vi "subvi_jenoptik_monotonize.vi"(1 "Array":dbl[](array[numeric]) format="%.2f") -> (0 "phase":dbl[](array[numeric]) format="%.2f")   [LabVIEW 2020]
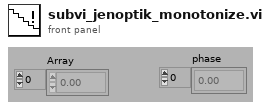
[diagram p1: front panel]
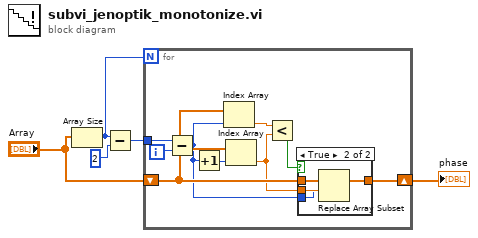
[diagram p0: block diagram]
diagram:
  n1 = Array Size(array="Array") -> (size(s)=w3:i32)
  n2 = Subtract(x=w3, y=2) -> (x-y=w2:i32)
  n3 = for {
    N: w3 -> [_]
    shift-right: [w14] -> w4
    shift-left: "Array" -> [w10]
    tunnel: w2 -> [w13]
    i -> [w12]
    n4 = Subtract(x=w13, y=w12) -> (x-y=w6:i32)
    n5 = Increment(x=w6) -> (x+1=w11:i32)
    n6 = Index Array(array=w10, index=w6) -> (element=w9:dbl)
    n7 = Index Array(array=w10, index=w11) -> (element=w7:dbl)
    n8 = Less?(x=w9, y=w7) -> (x < y?=w8:bool)
    n9 = case shown="True" w8 {
      tunnel: [w15 w19] -> w14
      tunnel: w10 -> [w15 w18]
      tunnel: w7 -> [_ w17]
      tunnel: w6 -> [_ w16]
      frame False {
      }
      frame True {
        n10 = Replace Array Subset(array=w18, new element=w17, index=w16) -> (w19:dbl[])
      }
    }
  }
  "phase" <- w4
